vi "Settings (class variable).vi"() -> ()   [LabVIEW 2016, in "Error Manager.lvlib" / "Settings.lvclass"]
uses:
  Settings.lvclass
panel:
  in  "Settings":refnum<class "Settings.lvclass">
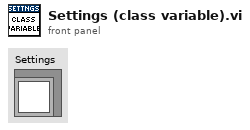
[diagram p1: front panel]
diagram:
